vi "deleteNode.vi"(8 "error in (no error)":errorcluster, 9 "elementForDeletion":string="channel_number type=\"digital\"", 10 "searchInElement":string="/device_settings/analog_output name=\"Ao32\"", 11 "xmlNode in":refnum<class "xmlNode.lvclass">) -> (0 "error out":errorcluster, 2 "xmlNodeReplacement":refnum<class "xmlNode.lvclass">, 3 "xmlNode out":refnum<class "xmlNode.lvclass">)   [LabVIEW 2011, in "Tools.lvlib" / "xml.lvlib" / "xmlNode.lvclass"]
doc: "deletes the xml node from the struture"
uses:
  xmlNode.lvclass
  XmlParser.lvclass
panel:
  out "String":string
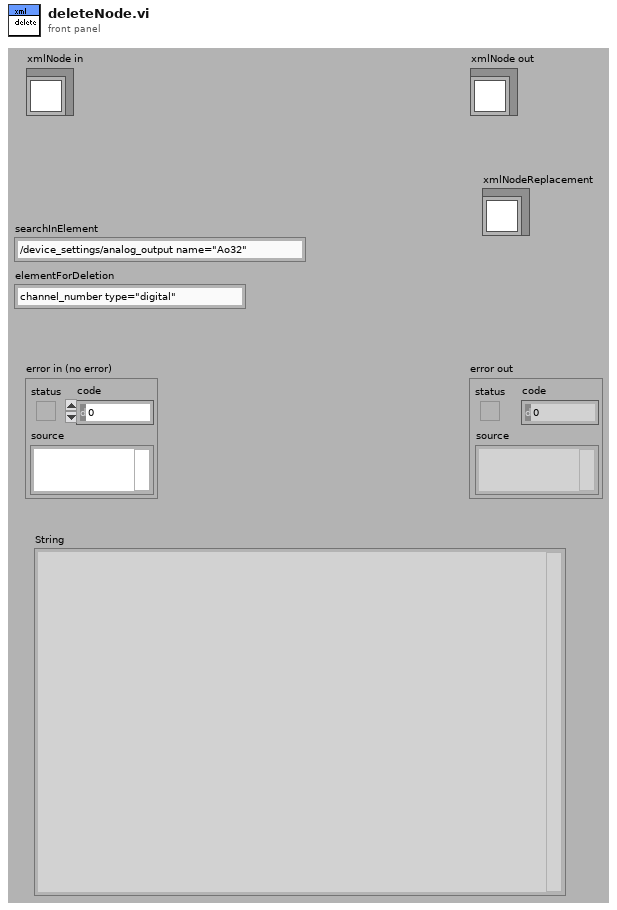
[diagram p1: front panel]
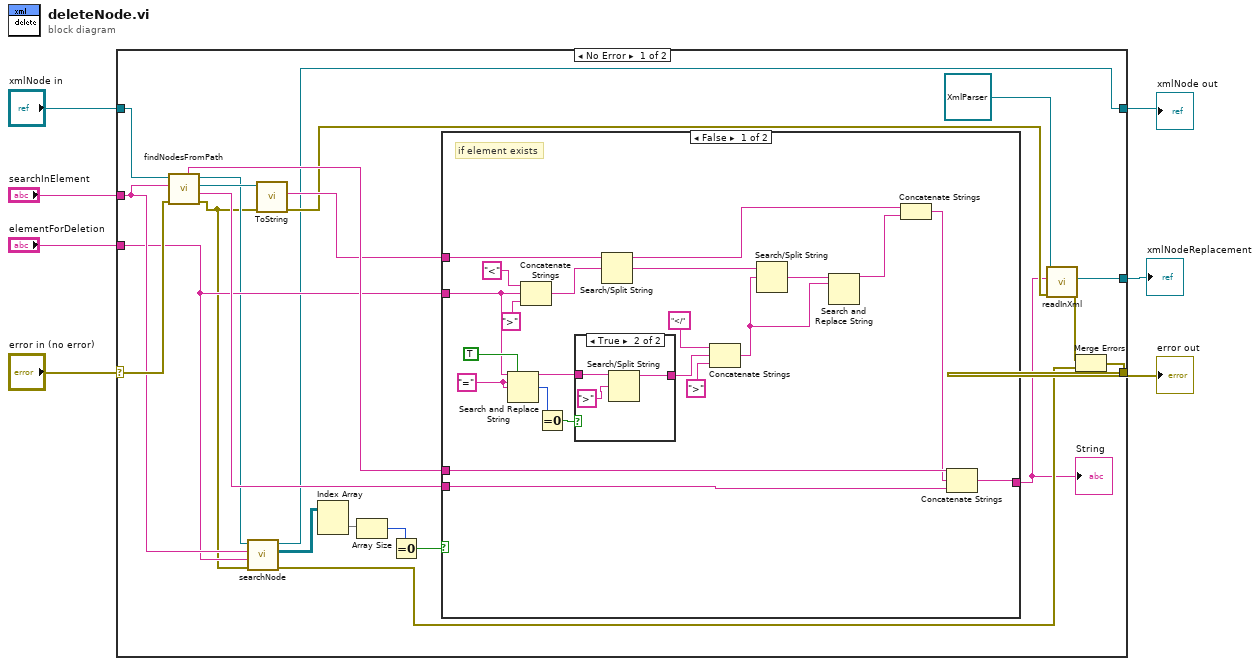
[diagram p0: block diagram]
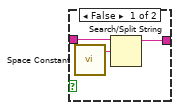
[diagram p2: hidden frame]
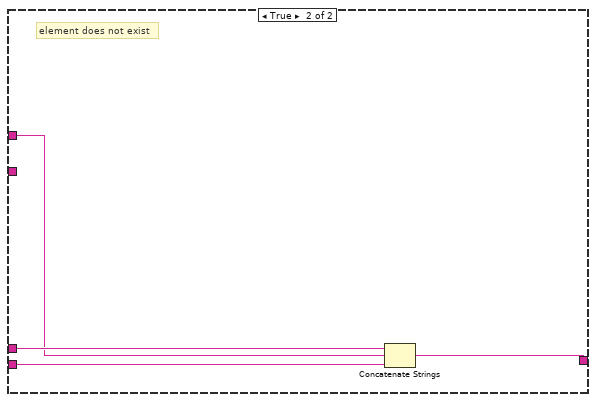
[diagram p3: hidden frame]
diagram:
  n1 = case shown="No Error" "error in (no error)" {
    selector: "error in (no error)" -> [w28 w63]
    tunnel: [w11 w63] -> w6
    tunnel: [w9 w62] -> w4
    tunnel: "xmlNode in" -> [w20 w62]
    tunnel: "searchInElement" -> [w19 _]
    tunnel: "elementForDeletion" -> [w18 _]
    tunnel: [w10 _] -> w1
    frame No Error {
      n2 = call "findNodesFromPath.vi"("error in (no error)"=w28, "searchInElement"=w19, "xmlNode in"=w20) -> ("error out"=w14:errorcluster, "rest of xml"=w25:string, "xmlNode"=w27:refnum<class "xmlNode.lvclass">, "xmlNode out"=w17:refnum<class "xmlNode.lvclass">, "xml before"=w26:string)  [unwired: 4 in]
      n3 = call-dynamic "searchNode.vi"("error in (no error)"=w14, "searchElementName"=w18, "searchElementIn"=w19, "xmlNode in"=w17) -> ("error out"=w12:errorcluster, "arrayXmlNodes"=w15:refnum<class "xmlNode.lvclass">[][], "xmlNode out"=w9:refnum<class "xmlNode.lvclass">)  [unwired: 5 in]
      n4 = call-dynamic "ToString.vi"("error in (no error)"=w14, "xmlNode in"=w27) -> ("error out"=w21:errorcluster, "xml"=w24:string)  [unwired: 7 in, 1 out]
      n5 = Index Array(array=w15) -> (element=w16:refnum<class "xmlNode.lvclass">[])  [unwired: 2 in]
      n6 = Array Size(array=w16) -> (size(s)=w29:i32)
      n7 = Equal To 0?(x=w29) -> (x = 0?=w23:bool)
      n8 = case shown="False" w23 {
        tunnel: w26 -> [w51 w61]
        tunnel: w25 -> [w50 w60]
        tunnel: w24 -> [w37 w58]
        tunnel: w18 -> [w36 _]
        tunnel: [w35 w59] -> w8
        frame False {
          w46 = "="
          # "if element exists"
          n9 = Search and Replace String(replace all?=TRUE, input string=w36, search string=w46, replace string=w46) -> (result string=w43:string, number of replacements=w45:i32)  [unwired: 4 in, 2 out]
          n10 = Concatenate Strings("<", w36, ">") -> (w48:string)
          n11 = Equal To 0?(x=w45) -> (x = 0?=w44:bool)
          n12 = case shown="True" w44 {
            tunnel: w43 -> [w54 w57]
            tunnel: [w52 w55] -> w40
            frame False {
              n13 = call <vilib>:"Space Constant.vi"() -> ("String"=w53:string)
              n14 = Search/Split String(string=w54, search string/char (-)=w53) -> (substring before match=w52:string)  [unwired: 1 in, 2 out]
            }
            frame True {
              n15 = Search/Split String(string=w57, search string/char (-)=">") -> (substring before match=w55:string)  [unwired: 1 in, 2 out]
            }
          }
          n16 = Search/Split String(string=w37, search string/char (-)=w48) -> (substring before match=w47:string, match + rest of string=w38:string)  [unwired: 1 in, 1 out]
          n17 = Concatenate Strings("</", w40, ">") -> (w32:string)
          n18 = Search/Split String(string=w38, search string/char (-)=w32) -> (match + rest of string=w33:string)  [unwired: 1 in, 2 out]
          n19 = Search and Replace String(input string=w33, search string=w32) -> (result string=w31:string)  [unwired: 6 in, 3 out]
          n20 = Concatenate Strings(w47, w31) -> (w30:string)
          n21 = Concatenate Strings(w51, w30, w50) -> (w35:string)
        }
        frame True {
          # "element does not exist"
          n22 = Concatenate Strings(w61, w58, w60) -> (w59:string)
        }
      }
      "String" <- w8
      n23 = call "readInXml.vi"("error in (no error)"=w21, "xmlString"=w8, "XmlParser in"=refnum<class "XmlParser.lvclass"> refnum ("Tools.lvlib:xml.lvlib:XmlParser.lvclass")) -> ("error out"=w13:errorcluster, "xmlNode"=w10:refnum<class "xmlNode.lvclass">)  [unwired: 6 in, 1 out]
      n24 = Merge Errors(w13, w12) -> (w11:errorcluster)
    }
    frame Error {
    }
  }
  "error out" <- w6
  "xmlNode out" <- w4
  "xmlNodeReplacement" <- w1
